vi "Class_ModuleName.vi"() -> (3 "Module Name":string)   [LabVIEW 2020]
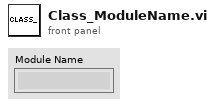
[diagram p1: front panel]
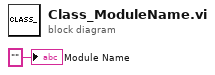
[diagram p0: block diagram]
diagram:
  "Module Name" <- ""
